vi "Create (Length).vi"(8 "error in (no error)":errorcluster, 11 "String value in":i8[](array[numeric])) -> (0 "error out":errorcluster, 3 "String out":refnum<class "String.lvclass">)   [LabVIEW 2012, in "MDSplus.lvlib" / "String.lvclass"]
uses:
  <vilib>/MDSplus/Classes/Data_Class/Scalar_Class/String_Class/String.lvclass
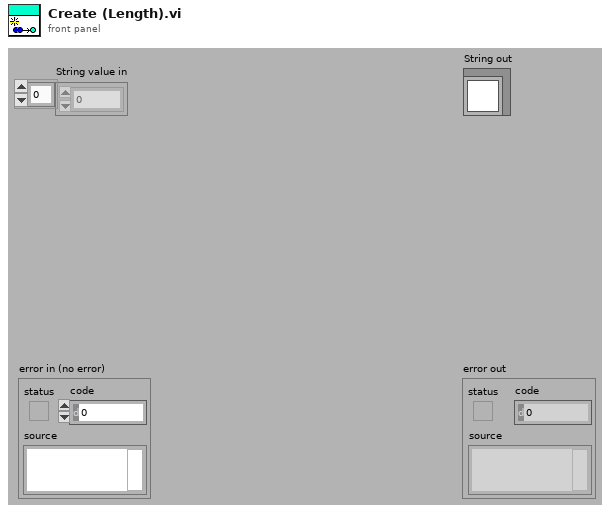
[diagram p1: front panel]
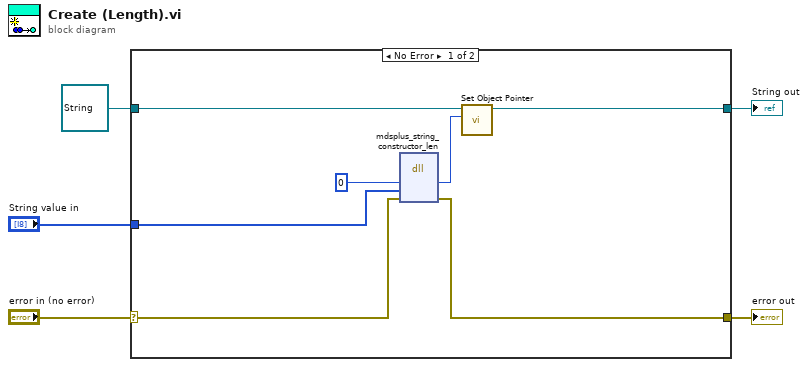
[diagram p0: block diagram]
diagram:
  n1 = case shown="No Error" "error in (no error)" {
    selector: "error in (no error)" -> [w10 w14]
    tunnel: [w6 w14] -> w4
    tunnel: [w7 w13] -> w2
    tunnel: refnum<class "String.lvclass"> refnum ("Float32 in") -> [w8 w13]
    tunnel: "String value in" -> [w9 _]
    frame No Error {
      n2 = dll-call lib="MDSobjectsLVShr" fn="mdsplus_string_constructor_len"("lvStringPtrOut"=i64 0 ("lvTreePtr"), "lvByteArrHdlIn"=w9, "error"=w10) -> ("lvStringPtrOut"=w11:i64, "error"=w6:errorcluster)  [unwired: 5 in, 2 out]
      n3 = call-dynamic "Set Object Pointer.vi"("Object Pointer"=w11, "Data in"=w8) -> ("Data out"=w7:refnum<class "String.lvclass">)  [unwired: 9 in]
    }
    frame Error {
    }
  }
  "error out" <- w4
  "String out" <- w2
